vi "Worker to Revert Config.vi"(8 "Error In":errorcluster, 11 "Revert Worker Config":T1={"Job Queue"=refnum, "Job Done Queue"=refnum, "Source Directory"=path "", "Unzip Directory"=path "", "Backsave Directory"=path "", "Output Directory"=path "", "Source File Name"="", "Output Path"="", "LabVIEW Version"=enum."13.0", "Archive Directory"=path ""}) -> (0 "Error Out":errorcluster, 2 "Revert Config":T3={"Revert Paths"={"Archive Path"=path "D:/workspace/revert/todo/todo.zip", "Unzip Directory"=path "D:/workspace/revert/unzip", "Backsave Directory"=path "D:/workspace/revert/backsave", "Output Archive"=path "D:/workspace/revert/backsave", "Backsave Common Directory"=path "D:/workspace/revert/backsave"}, "LabVIEW Files"={"Projects"=[], "Libraries"=[], "Classes"=[], "XControls"=[], "VIs and Controls"=[], "Non LV Files"=[]}, "LabVIEW Version"=enum."8.0"}, 3 "Revert Worker Config":T1={"Job Queue"=refnum, "Job Done Queue"=refnum, "Source Directory"=path "", "Unzip Directory"=path "", "Backsave Directory"=path "", "Output Directory"=path "", "Source File Name"="", "Output Path"="", "LabVIEW Version"=enum."13.0", "Archive Directory"=path ""})   [LabVIEW 2013, in "LVH-Revert.lvlib"]
uses:
  <vilib>/LabVIEW Hacker/Revert/LVH-Revert.lvlib
  <vilib>/LabVIEW Hacker/Revert/Private/Revert Worker Config.ctl
  <vilib>/National Instruments/NI Amazon Web Services (AWS) Toolkit for LabVIEW/SQS/VI Source/AWS SQS Class/AWS_SQS.lvclass
  <vilib>/National Instruments/NI Amazon Web Services (AWS) Toolkit for LabVIEW/AWS Core Lib/VI Source/Canonicals/AWS_Core Canonical Credentials/Canonical Credentials.lvclass
  <vilib>/National Instruments/NI Amazon Web Services (AWS) Toolkit for LabVIEW/AWS Core Lib/VI Source/Canonicals/AWS_Core Canonical Required Parameters/Canonical Required Parameters.lvclass
  <vilib>/National Instruments/NI Amazon Web Services (AWS) Toolkit for LabVIEW/SQS/VI Source/Canonicals/Canonical CreateQueue/Canonical CreateQueue.lvclass
  <vilib>/National Instruments/NI Amazon Web Services (AWS) Toolkit for LabVIEW/SQS/VI Source/Canonicals/Canonical ListQueues/Canonical ListQueues.lvclass
  <vilib>/National Instruments/NI Amazon Web Services (AWS) Toolkit for LabVIEW/SQS/VI Source/Canonicals/Canonical AddPermission/Canonical AddPermission.lvclass
  <vilib>/National Instruments/NI Amazon Web Services (AWS) Toolkit for LabVIEW/SQS/VI Source/Canonicals/Canonical ChangeMessageVisibility/Canonical ChangeMessageVisibility.lvclass
  <vilib>/National Instruments/NI Amazon Web Services (AWS) Toolkit for LabVIEW/SQS/VI Source/Canonicals/Canonical ChangeMessageVisibilityBatch/Canonical ChangeMessageVisibilityBatch.lvclass
  <vilib>/National Instruments/NI Amazon Web Services (AWS) Toolkit for LabVIEW/SQS/VI Source/Canonicals/Canonical DeleteMessage/Canonical DeleteMessage.lvclass
  <vilib>/National Instruments/NI Amazon Web Services (AWS) Toolkit for LabVIEW/SQS/VI Source/Canonicals/Canonical DeleteMessageBatch/Canonical DeleteMessageBatch.lvclass
  <vilib>/National Instruments/NI Amazon Web Services (AWS) Toolkit for LabVIEW/SQS/VI Source/Canonicals/Canonical GetQueueAttributes/Canonical GetQueueAttributes.lvclass
  <vilib>/National Instruments/NI Amazon Web Services (AWS) Toolkit for LabVIEW/SQS/VI Source/Canonicals/Canonical GetQueueUrl/Canonical GetQueueUrl.lvclass
  <vilib>/National Instruments/NI Amazon Web Services (AWS) Toolkit for LabVIEW/SQS/VI Source/Canonicals/Canonical ReceiveMessage/Canonical ReceiveMessage.lvclass
  <vilib>/National Instruments/NI Amazon Web Services (AWS) Toolkit for LabVIEW/SQS/VI Source/Canonicals/Canonical RemovePermission/Canonical RemovePermission.lvclass
  <vilib>/National Instruments/NI Amazon Web Services (AWS) Toolkit for LabVIEW/SQS/VI Source/Canonicals/Canonical SendMessage/Canonical SendMessage.lvclass
  <vilib>/National Instruments/NI Amazon Web Services (AWS) Toolkit for LabVIEW/SQS/VI Source/Canonicals/Canonical SendMessageBatch/Canonical SendMessageBatch.lvclass
  <vilib>/National Instruments/NI Amazon Web Services (AWS) Toolkit for LabVIEW/SQS/VI Source/Canonicals/Canonical SetQueueAttributes/Canonical SetQueueAttributes.lvclass
  <vilib>/LabVIEW Hacker/LVH-Toolbox/Common/Private/Type Defs/LabVIEW Version.ctl
  <vilib>/LabVIEW Hacker/Revert/Type Defs/Revert Config.ctl
  <vilib>/LabVIEW Hacker/Revert/Type Defs/Paths.ctl
  <vilib>/LabVIEW Hacker/Revert/Type Defs/LabVIEW Files.ctl
  <vilib>/LabVIEW Hacker/LVH-Toolbox/Common/LVH-Common.lvlib
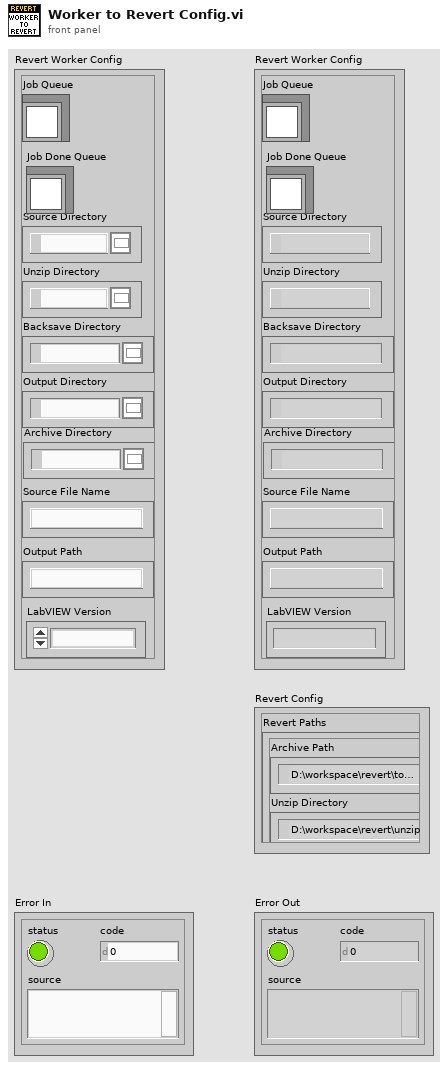
[diagram p1: front panel]
types:
  T1 = typedef "LVH-Revert.lvlib/Revert Worker Config.ctl" = cluster{"Job Queue":refnum<class "AWS_SQS.lvclass">, "Job Done Queue":refnum<class "AWS_SQS.lvclass">, "Source Directory":path, "Unzip Directory":path, "Backsave Directory":path, "Output Directory":path, "Source File Name":string, "Output Path":string, "LabVIEW Version":T2, "Archive Directory":path}
  T2 = typedef "LVH-Toolbox.lvlib/LVH-Common.lvlib/LabVIEW Version.ctl" = enum16{"8.0", "8.2", "8.6", "9.0", "10.0", "11.0", "12.0", "13.0"}
  T3 = typedef "LVH-Revert.lvlib/Revert Config.ctl" = cluster{"Revert Paths":T4, "LabVIEW Files":T5, "LabVIEW Version":T2}
  T4 = typedef "LVH-Revert.lvlib/Paths.ctl" = cluster{"Archive Path":path, "Unzip Directory":path, "Backsave Directory":path, "Output Archive":path, "Backsave Common Directory":path}
  T5 = typedef "LVH-Revert.lvlib/LabVIEW Files.ctl" = cluster{"Projects":path[], "Libraries":path[], "Classes":path[], "XControls":path[], "VIs and Controls":path[], "Non LV Files":path[]}
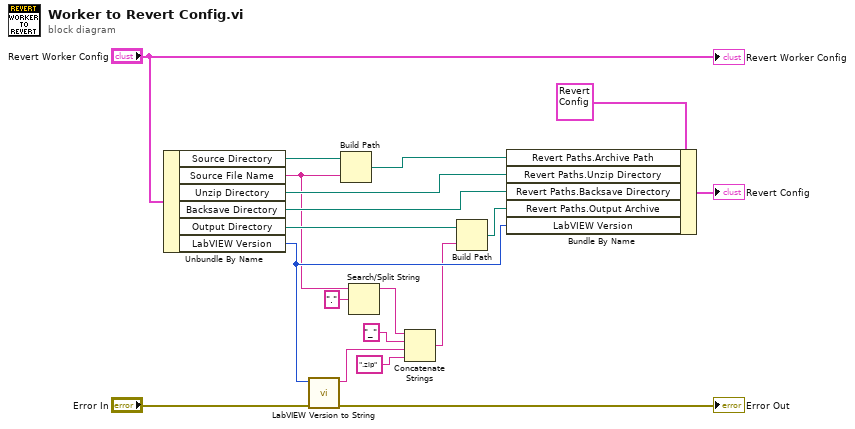
[diagram p0: block diagram]
diagram:
  n1 = Unbundle By Name("Revert Worker Config") -> ("Source Directory"=w16:path, "Source File Name"=w3:string, "Unzip Directory"=w14:path, "Backsave Directory"=w13:path, "Output Directory"=w12:path, "LabVIEW Version"=w8:T2)
  n2 = call <vilib>:"LabVIEW Version to String.vi"("Error In"="Error In", "LabVIEW Version"=w8) -> ("Error Out"=→"Error Out":errorcluster, "LabVIEW Version"=w7:string)  [unwired: 8 in]
  n3 = Build Path(base path=w16, name or relative path=w3) -> (appended path=w15:path)
  n4 = Search/Split String(string=w3, search string/char (-)=".") -> (substring before match=w1:string)  [unwired: 1 in, 2 out]
  n5 = Concatenate Strings(w1, "_" ("string"), w7, ".zip" ("string")) -> (w6:string)
  n6 = Build Path(base path=w12, name or relative path=w6) -> (appended path=w5:path)
  n7 = Bundle By Name(cluster=T3 {"Revert Paths"={"Archive Path"=path "D:/workspace/revert/todo/todo.zip", "Unzip Directory"=path "D:/workspace/revert/unzip", "Backsave Directory"=path "D:/workspace/revert/backsave", "Output Archive"=path "D:/workspace/revert/output/out.zip", "Backsave Common Directory"=path "D:/workspace/revert/backsave"}, "LabVIEW Files"={"Projects"=[], "Libraries"=[], "Classes"=[], "XControls"=[], "VIs and Controls"=[], "Non LV Files"=[]}, "LabVIEW Version"=enum."8.0"} ("Revert Config"), "Revert Paths.Archive Path"=w15, "Revert Paths.Unzip Directory"=w14, "Revert Paths.Backsave Directory"=w13, "Revert Paths.Output Archive"=w5, "LabVIEW Version"=w8) -> (→"Revert Config":T3)
  "Revert Worker Config" <- "Revert Worker Config"
